vi "Utility Parse Fault Status.vi"(8 "error in (no error)":errorcluster, 11 "Fault Status Response":string) -> (0 "error out":errorcluster, 3 "Fault Status Cluster out":T1)   [LabVIEW 2020, in "ChromTech Series III Pump.lvlib"]
uses:
  <instrlib>/RxnRover/ChromtechSeriesIIIDriver/ChromTech Series III Pump.lvlib
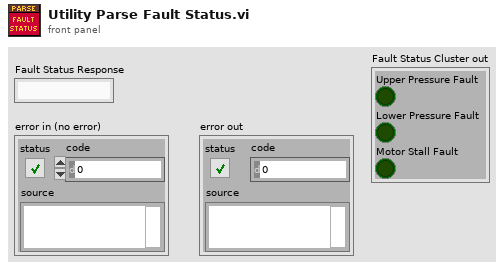
[diagram p1: front panel]
types:
  T1 = cluster{"Upper Pressure Fault":bool, "Lower Pressure Fault":bool, "Motor Stall Fault":bool}
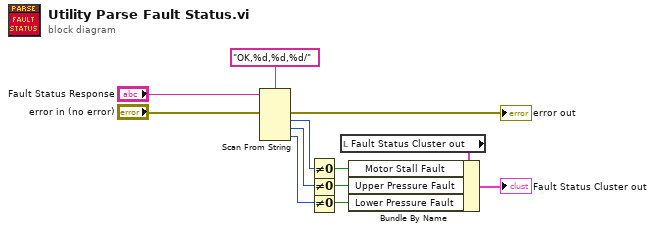
[diagram p0: block diagram]
diagram:
  n1 = Scan From String(format string="OK,%d,%d,%d/", input string="Fault Status Response", error in="error in (no error)") -> (error out=→"error out":errorcluster, output 1=w3:i32, output 2=w2:i32, output 3=w1:i32)  [unwired: 4 in, 2 out]
  n2 = Not Equal To 0?(x=w3) -> (x != 0?=w6:bool)
  n3 = Not Equal To 0?(x=w2) -> (x != 0?=w5:bool)
  n4 = Not Equal To 0?(x=w1) -> (x != 0?=w4:bool)
  n5 = local read "Fault Status Cluster out"() -> (w8:T1)
  n6 = Bundle By Name(cluster=w8, "Motor Stall Fault"=w6, "Upper Pressure Fault"=w5, "Lower Pressure Fault"=w4) -> (→"Fault Status Cluster out":T1)
